vi "PH_TKTDS-30xx.Init.vi"(0 "i ref in":refnum<vi>, 5 "error in (no error)":errorcluster) -> (14 "i ref out":refnum<vi>, 19 "error out":errorcluster)   [LabVIEW 2014, in "PH_TKTDS-30xx.lvlib"]
doc: "Initializes the connection to the hardware and queries the errors which are written to own attributes. The \"connection established\" flag is set to true in case of no error."
uses:
  PH_TKTDS-30xx.lvlib
  instr.lib/TKDS3032-PHELIX/tktds3032-PHELIX - Driver np.lvlib
  PH_Basics/PH_Common/PH_Common.lvlib
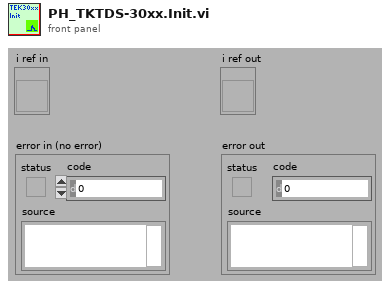
[diagram p1: front panel]
types:
  T1 = typedef "PH_TKTDS-30xx.lvlib/PH_TKTDS-30xx.i attribute.ctl" = cluster{"Default VISA Resource":string, "VISA Resource Name":refnum<visa-resource-name>, "Revision":cluster{"Instrument Driver":string, "Instrument Firmware":string}, "Selftest":cluster{"Result":u32, "Message":string}, "Channels":T2[], "Trigger Configuration":T3, "Acquisition Configuration":T4, "Fetched Waveforms":T5[], "GUI Refs":T6, "GUI Refs Channels":refnum<vi>[], "State":T7, "Error Message":string, "Allow Prdc Loop?":bool}
  T2 = typedef "PH_TKTDS-30xx.lvlib/PH_TKTDS-30xx.Channel Config.ctl" = cluster{"Channel Name":string, "Input Impedance":string, "Max Input Frequency":string, "Vertical Coupling":i32, "Channel Enabled":bool, "Probe Attenuation":dbl, "Vertical Range":dbl, "Vertical Offset":dbl}
  T3 = typedef "PH_TKTDS-30xx.lvlib/PH_TKTDS-30xx.Trigger Config.ctl" = cluster{"Source":string, "Slope":i32, "Level [V]":dbl}
  T4 = typedef "PH_TKTDS-30xx.lvlib/PH_TKTDS-30xx.Acquisition Config.ctl" = cluster{"Time base":dbl, "Record Length":u16, "Start Time":dbl, "Type":i32, "Continuous":bool}
  T5 = typedef "PH_TKTDS-30xx.lvlib/PH_TKTDS-30xx.fetched Waveform.ctl" = cluster{"Source":string, "Actual Points":u32, "Initial X":dbl, "X Increment":dbl, "Waveform Array":dbl[]}
  T6 = typedef "PH_TKTDS-30xx.lvlib/PH_TKTDS-30xx.GUI Refs.ctl" = cluster{"Trigger":refnum<vi>, "Acquisition":refnum<vi>, "Graph":refnum<vi>, "State":refnum<vi>, "Delete":refnum<vi>, "Channel to be positioned":refnum<vi>, "Postion":refnum<vi>, "Display Intensity":refnum<vi>, "VISA Resource":refnum<vi>}
  T7 = typedef "PH_StatusHandler.lvlib/PH_StatusHandler.Status.ctl" = i16
  T8 = cluster{"Baud Rate (9600)":u32, "Flow Control (RTS/CTS)":u16, "Data Bits (8)":u16}
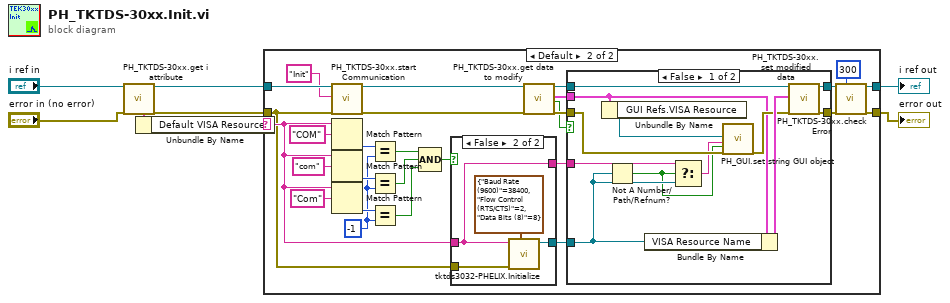
[diagram p0: block diagram]
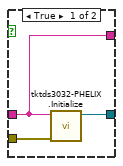
[diagram p3: hidden frame]
diagram:
  n1 = call "PH_TKTDS-30xx.get i attribute.vi"("i ref in"="i ref in", "error in (no error)"="error in (no error)") -> ("i ref out"=w7:refnum<vi>, "i attribute"=w3:T1, "error out"=w5:errorcluster)  [unwired: 15 in]
  n2 = Unbundle By Name(w3) -> ("Default VISA Resource"=w4:string)
  n3 = case shown="Default" w4 {
    selector: w4 -> [_ w38]
    tunnel: w5 -> [w10 w15]
    tunnel: [w10 w19] -> w6
    tunnel: w7 -> [w9 w17]
    tunnel: [w9 w21] -> w8
    frame "", "N/A" {
    }
    frame Default {
      w27 = -1 ("y")
      n4 = call "PH_TKTDS-30xx.start Communication.vi"("i ref in"=w17, "Action"="Init", "error in"=w15) -> ("i ref out"=w16:refnum<vi>, "error out"=w14:errorcluster)  [unwired: 15 in]
      n5 = Match Pattern(string=w38, regular expression="COM") -> (offset past match=w30:i32)  [unwired: 1 in, 3 out]
      n6 = Match Pattern(string=w38, regular expression="com") -> (offset past match=w29:i32)  [unwired: 1 in, 3 out]
      n7 = Match Pattern(string=w38, regular expression="Com") -> (offset past match=w28:i32)  [unwired: 1 in, 3 out]
      n8 = Equal?(x=w30, y=w27) -> (x = y?=w26:bool)
      n9 = Equal?(x=w29, y=w27) -> (x = y?=w25:bool)
      n10 = Equal?(x=w28, y=w27) -> (x = y?=w24:bool)
      n11 = Compound Arithmetic op=AND(w26, w25, w24) -> (w23:bool)
      n12 = case shown="False" w23 {
        tunnel: [w41 w45] -> w18
        tunnel: w15 -> [w40 w44]
        tunnel: w38 -> [w39 w42]
        tunnel: [w39 w42] -> w11
        frame True {
          n13 = call "tktds3032-PHELIX.Initialize.vi"("error in (no error)"=w40, "VISA Resource Name"=w39) -> ("VISA Resource Name Out"=w41:refnum<visa-resource-name>)  [unwired: 8 in, 1 out]
        }
        frame False {
          n14 = call "tktds3032-PHELIX.Initialize.vi"("Serial Settings"=T8 {"Baud Rate (9600)"=38400, "Flow Control (RTS/CTS)"=2, "Data Bits (8)"=8}, "error in (no error)"=w44, "VISA Resource Name"=w42) -> ("VISA Resource Name Out"=w45:refnum<visa-resource-name>)  [unwired: 7 in, 1 out]
        }
      }
      n15 = call "PH_TKTDS-30xx.get data to modify.vi"("i ref in"=w16, "error in (no error)"=w14) -> ("i ref out"=w36:refnum<vi>, "i attribute"=w34:T1, "timed out"=w35:bool, "error out"=w37:errorcluster)  [unwired: 14 in]
      n16 = case shown="False" w35 {
        tunnel: [w57 w58] -> w20
        tunnel: w37 -> [w56 w58]
        tunnel: w36 -> [w55 w59]
        tunnel: [w54 w59] -> w22
        tunnel: w34 -> [w51 _]
        tunnel: w18 -> [w47 _]
        tunnel: w11 -> [w49 _]
        frame False {
          n17 = Unbundle By Name(w51) -> ("GUI Refs.VISA Resource"=w50:refnum<vi>)
          n18 = Not A Number/Path/Refnum?(number/path/refnum=w47) -> (NaN/Path/Refnum?=w46:bool)
          n19 = Bundle By Name(cluster=w51, "VISA Resource Name"=w47) -> (w53:T1)
          n20 = Select(t=w49, s=w46, f=w47) -> (s? t:f=w48:string)
          n21 = call "PH_GUI.set string GUI object.vi"("GUI object Ref"=w50, "Text"=w48, "Blinking? (false)"=w46, "error in"=w56) -> ("error out"=w52:errorcluster)  [unwired: 15 in]
          n22 = call "PH_TKTDS-30xx.set modified data.vi"("i ref in"=w55, "i attribute"=w53, "error in (no error)"=w52) -> ("i ref out"=w54:refnum<vi>, "error out"=w57:errorcluster)  [unwired: 15 in]
        }
        frame True {
        }
      }
      n23 = call "PH_TKTDS-30xx.check Error.vi"("i ref in"=w22, "Waiting Time [ms]"=u32 300, "error in"=w20) -> ("i ref out"=w21:refnum<vi>, "error out"=w19:errorcluster)  [unwired: 15 in]
    }
  }
  "i ref out" <- w8
  "error out" <- w6
